vi "Parse Cash Data.vi"(11 "Tournament Data In":string) -> (3 "Cash Data":T1)   [LabVIEW 2020]
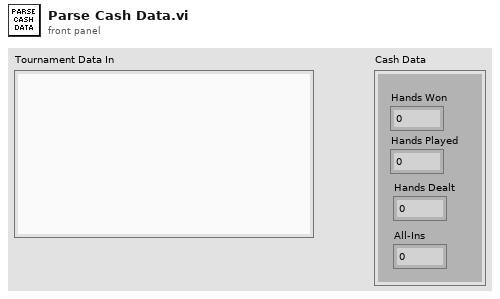
[diagram p1: front panel]
types:
  T1 = cluster{"Hands Won":i32, "Hands Played":i32, "Hands Dealt":i32, "All-Ins":i32}
  T2 = cluster{"Stat Value":i32, "Stat Value":i32, "Stat Value":i32, "Stat Value":i32}
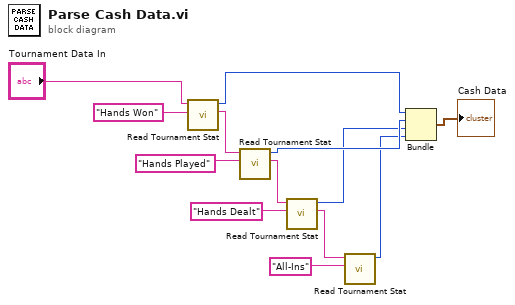
[diagram p0: block diagram]
diagram:
  n1 = call "Read Tournament Stat.vi"("Stat Name"="Hands Won" ("Stat String"), "Tournament Data In in"="Tournament Data In") -> ("Remaining String Out"=w11:string, "Stat Value"=w5:i32)  [unwired: 8 in]
  n2 = call "Read Tournament Stat.vi"("Stat Name"="Hands Played" ("regular expression"), "Tournament Data In in"=w11) -> ("Remaining String Out"=w10:string, "Stat Value"=w4:i32)  [unwired: 8 in]
  n3 = call "Read Tournament Stat.vi"("Stat Name"="Hands Dealt" ("regular expression"), "Tournament Data In in"=w10) -> ("Remaining String Out"=w9:string, "Stat Value"=w3:i32)  [unwired: 8 in]
  n4 = call "Read Tournament Stat.vi"("Stat Name"="All-Ins" ("regular expression"), "Tournament Data In in"=w9) -> ("Stat Value"=w2:i32)  [unwired: 8 in, 1 out]
  n5 = Bundle("Stat Value"=w5, "Stat Value"=w4, "Stat Value"=w3, "Stat Value"=w2) -> (→"Cash Data":T2)  [unwired: 1 in]
